vi "2023 Begin Logic.vi"(1 "error in (no error)":errorcluster) -> (0 "error out":errorcluster)   [LabVIEW 2020]
uses:
  2023 Robot Global Data.vi
panel:
  out "robotID":string="981-2023"
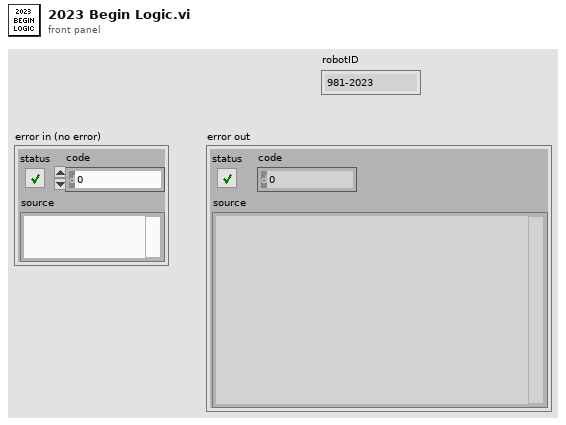
[diagram p1: front panel]
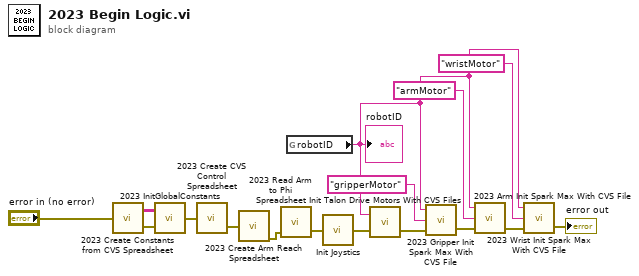
[diagram p0: block diagram]
diagram:
  n1 = call "2023 Create Constants from CVS Spreadsheet.vi"("error in"="error in (no error)") -> ("localConstantSpreadSheet"=w13:string[][], "error out"=w14:errorcluster)
  n2 = call "2023 InitGlobalConstants.vi"("error in (no error)"=w14, "localConstantSpreadSheet"=w13) -> ("error out"=w15:errorcluster)
  n3 = call "2023 Create CVS Control Spreadsheet.vi"("error in"=w15) -> ("error out"=w3:errorcluster)  [unwired: 1 out]
  n4 = call "2023 Create Arm Reach Spreadsheet.vi"("error in"=w3) -> ("error out"=w2:errorcluster)  [unwired: 3 out]
  n5 = call "2023 Read Arm to Phi Spreadsheet.vi"("error in"=w2) -> ("error out"=w1:errorcluster)  [unwired: 2 in, 1 out]
  n6 = global read "2023 Robot Global Data.vi" "robotID"() -> (w5:string)
  "robotID" <- w5
  n7 = call "Init Joystics.vi"("error in"=w1) -> ("error out"=w9:errorcluster)
  n8 = call "Init Talon Drive Motors With CVS Files.vi"("error in"=w9, "Robot ID"=w5) -> ("error out"=w8:errorcluster)  [unwired: 1 out]
  n9 = call "2023 Gripper Init Spark Max With CVS File.vi"("error in"=w8, "Motor ID"="gripperMotor", "Robot ID"=w5) -> ("error out"=w11:errorcluster)  [unwired: 1 out]
  n10 = call "2023 Arm Init Spark Max With CVS File.vi"("error in"=w11, "Motor ID"="armMotor", "Robot ID"=w5) -> ("error out"=w7:errorcluster)  [unwired: 1 in, 1 out]
  n11 = call "2023 Wrist Init Spark Max With CVS File.vi"("error in"=w7, "Motor ID"="wristMotor", "Robot ID"=w5) -> ("error out"=→"error out":errorcluster)  [unwired: 1 out]
